vi "Query Asset Utilization.vi"(8 "Error In":errorcluster, 9 "Utilization Filter":string, 10 "Asset Filter":string, 11 "Session In":refnum<class "NI Skyline Configuration HTTP.lvclass">) -> (0 "Error Out":errorcluster, 2 "Asset Utilization":T1(array[cluster]), 3 "Session Out":refnum<class "NI Skyline Configuration HTTP.lvclass">)   [LabVIEW 2020]
uses:
  <vilib>/Skyline/Configuration/Configuration HTTP_class/NI Skyline Configuration HTTP.lvclass
  <vilib>/Skyline/Configuration/Configuration HTTP_class/NI Skyline Configuration HTTP.lvclass/NI Skyline Configuration HTTP.ctl
  <vilib>/Skyline/Configuration/Configuration HTTP_class/Read Server URL.vi
  <vilib>/httpClient/POSTBuffer.vi
  <vilib>/httpClient/LabVIEWHTTPClient.lvlib
  <vilib>/addons/_JKI.lib/Serialization/JSON/JKI JSON Serialization.lvlib
panel:
  out "Server URL":string
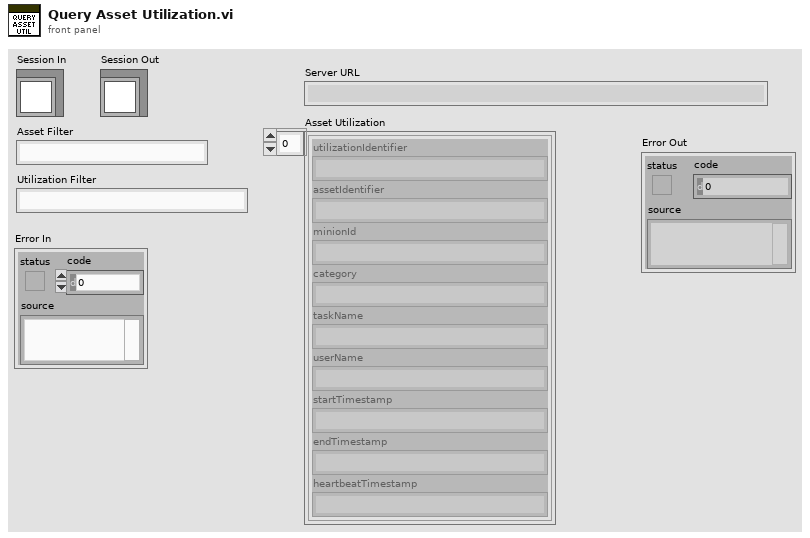
[diagram p1: front panel]
types:
  T1 = cluster{"utilizationIdentifier":string, "assetIdentifier":string, "minionId":string, "category":string, "taskName":string, "userName":string, "startTimestamp":string, "endTimestamp":string, "heartbeatTimestamp":string}[]
  T2 = cluster{"assetUtilizations":cluster{"utilizationIdentifier":string, "assetIdentifier":string, "minionId":string, "category":string, "taskName":string, "userName":string, "startTimestamp":string, "endTimestamp":string, "heartbeatTimestamp":string}[]}
  T3 = typedef "LabVIEWHTTPClient.lvlib/ClientHandle.ctl" = refnum<k1>
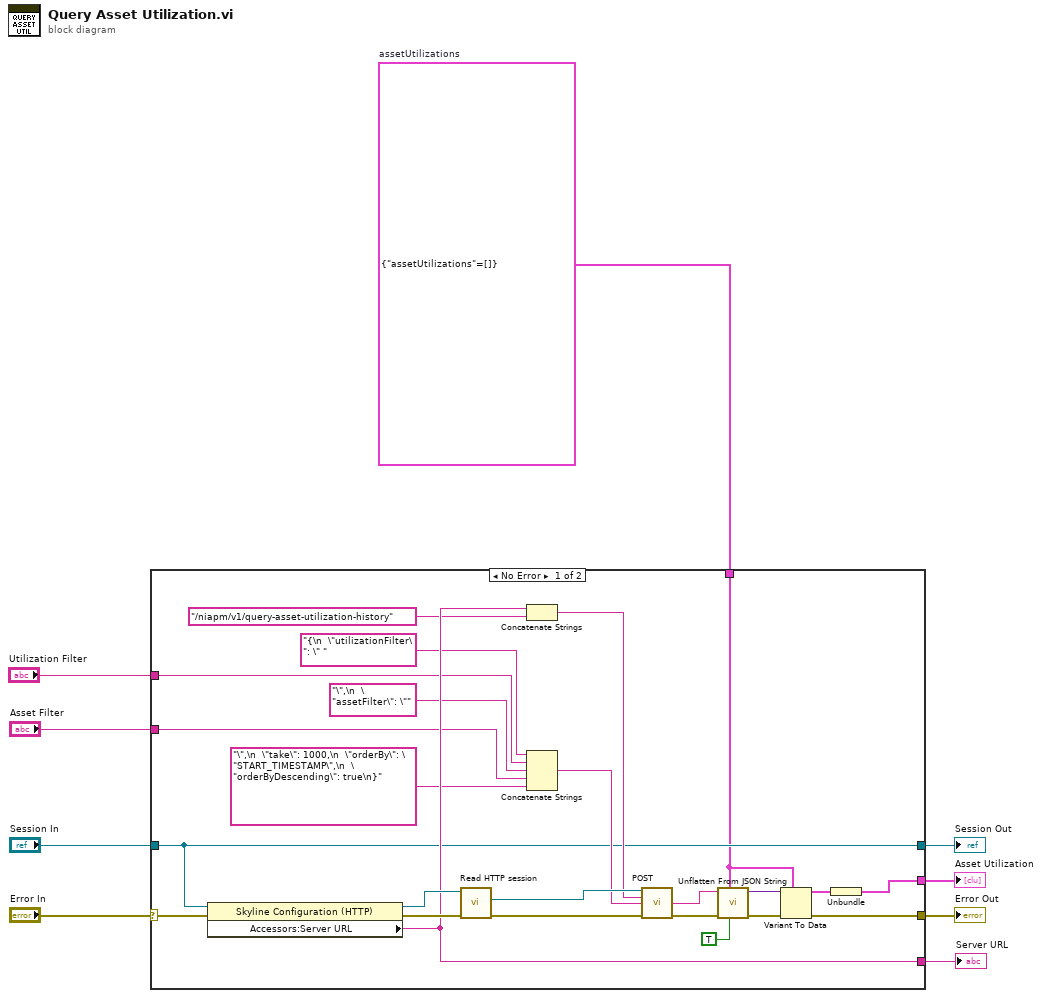
[diagram p0: block diagram]
diagram:
  w1 = T2 {"assetUtilizations"=[]}  # assetUtilizations
  n1 = case shown="No Error" "Error In" {
    selector: "Error In" -> [w13 w35]
    tunnel: [w29 _] -> w9
    tunnel: "Asset Filter" -> [w24 _]
    tunnel: "Utilization Filter" -> [w21 _]
    tunnel: "Session In" -> [w12 w34]
    tunnel: [w15 w35] -> w5
    tunnel: [w14 _] -> w4
    tunnel: [w12 w34] -> w2
    tunnel: w1 -> [w10 _]
    frame No Error {
      n2 = property class="Skyline Configuration (HTTP)"(reference=w12, error in=w13) -> (reference out=w32:refnum<class "NI Skyline Configuration HTTP.lvclass">, error out=w31:errorcluster, "Accessors:Server URL"=w29:string)
      n3 = call <vilib>:"Read HTTP session.vi"("error in (no error)"=w31, "HTTP configuration in"=w32) -> ("error out"=w30:errorcluster, "http session"=w33:T3)  [unwired: 7 in, 1 out]
      n4 = Concatenate Strings(w29, "/niapm/v1/query-asset-utilization-history" ("string")) -> (w28:string)
      n5 = Concatenate Strings("{\n  \"utilizationFilter\": \" " ("buffer"), w21, "\",\n  \"assetFilter\": \"" ("string"), w24, "\",\n  \"take\": 1000,\n  \"orderBy\": \"START_TIMESTAMP\",\n  \"orderByDescending\": true\n}" ("buffer")) -> (w25:string)
      n6 = call-poly <vilib>:"POST.vi"("client handle"=w33, "url"=w28, "buffer"=w25, "error in (no error)"=w30) -> ("body"=w11:string, "error out"=w20:errorcluster)  [unwired: 8 in, 2 out]
      n7 = call <vilib>:"Unflatten From JSON String.vi"("Nulls as Defaults (F)"=TRUE ("default null elements? (F)"), "Type and Defaults"=w10, "error in (no error)"=w20, "JSON String"=w11) -> ("error out"=w17:errorcluster, "Variant"=w18:variant)  [unwired: 6 in]
      n8 = Variant To Data(error in=w17, type=w10, Variant=w18) -> (data=w16:T2, error out=w15:errorcluster)
      n9 = Unbundle(w16) -> ("assetUtilizations"=w14:T1)
    }
    frame Error {
    }
  }
  "Server URL" <- w9
  "Error Out" <- w5
  "Asset Utilization" <- w4
  "Session Out" <- w2
